vi "alarm.vi"() -> ()   [LabVIEW 2025]
doc: "Author: Scott Hannahs <sth@magnet.fsu.edu>\n\nThis software is licensed for use under the “MIT License\"\nCopyright (c) 2025 Scott Hannahs, sth@sth@magnet.sthnet.net\n\nPermission is hereby granted, free of charge, to any person obtaining a copy of this software and associated documentation files (the \"Software\"), to deal in the Software without restriction, including without limitation the rights to use, copy, modify, merge, publish, distribute, sublicense, and/or sell copies of the Software, and to permit persons to whom the Software is furnished to do so, subject to the following conditions: The above copyright notice and this permission notice shall be included in all copies or substantial portions of the Software.\n\nTHE SOFTWARE IS PROVIDED \"AS IS\", WITHOUT WARRANTY OF ANY KIND, EXPRESS OR IMPLIED, INCLUDING BUT NOT LIMITED TO THE WARRANTIES OF MERCHANTABILITY, FITNESS FOR A PARTICULAR PURPOSE AND NONINFRINGEMENT. IN NO EVENT SHALL THE AUTHORS OR COPYRIGHT HOLDERS BE LIABLE FOR ANY CLAIM, DAMAGES OR OTHER LIABILITY, WHETHER IN AN ACTION OF CONTRACT, TORT OR OTHERWISE, ARISING FROM, OUT OF OR IN CONNECTION WITH THE SOFTWARE OR THE USE OR OTHER DEALINGS IN THE SOFTWARE."
panel:
  in  "up":bool
  in  "Stop Button":bool
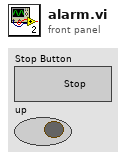
[diagram p1: front panel]
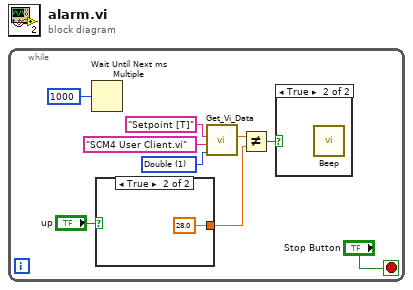
[diagram p0: block diagram]
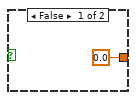
[diagram p2: hidden frame]
diagram:
  n1 = while {
    stop <- "Stop Button" stop-if-true
    w7 = u16 1 items=["String", "Double", "Boolean", "Variant"] ("Data Type")
    n2 = Wait Until Next ms Multiple(millisecond multiple=u32 1000) -> ()  [unwired: 1 out]
    n3 = case shown="True" "up" {
      tunnel: [0.0 ("y") 28.0 ("y")] -> w3
      frame False {
      }
      frame True {
      }
    }
    n4 = call "Get_Vi_Data.vi"("Data Type"=w7, "VI name"="SCM4 User Client.vi" ("Control Name"), "Control Name"="Setpoint [T]") -> ("Data (Double)"=w4:dbl)  [unwired: 4 in, 4 out]
    n5 = Not Equal?(x=w4, y=w3) -> (x != y?=w2:bool)
    n6 = case shown="True" w2 {
      frame False {
      }
      frame True {
        n7 = call <vilib>:"Beep.vi"() -> ()  [unwired: 12 in]
      }
    }
  }
